vi "SetConfig.vi"(8 "error in (no error)":errorcluster, 11 "reference in":refnum<class "Barcode_Reader_Dialog.lvclass">) -> (0 "error out":errorcluster, 3 "reference out":refnum<class "Barcode_Reader_Dialog.lvclass">)   [LabVIEW 2022 SP3, in "Barcode_Reader_Dialog.lvlib" / "Barcode_Reader_Dialog.lvclass"]
uses:
  Barcode_Reader_Dialog.lvclass
  Components/Barcode_Reader_Base.lvlibp/Barcode_Reader_Base.lvclass
  C:/Projects/Medulla/ViPER/Examples/Flux_Capacitor_Tester/Components/ViPER.lvlibp/ViPER.lvclass
  Components/ViPER.lvlibp/ViPER.lvclass
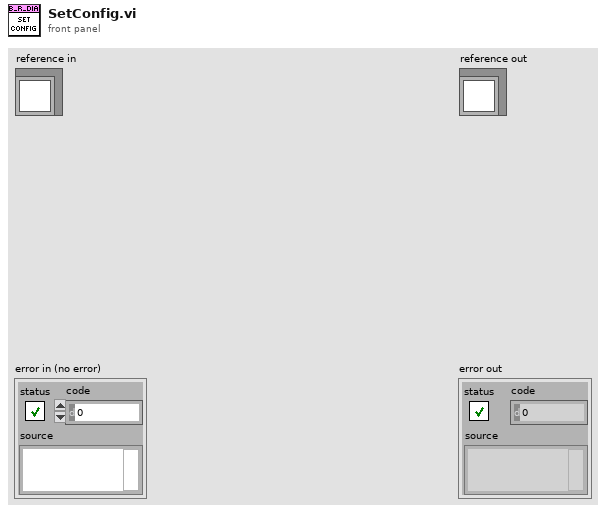
[diagram p1: front panel]
types:
  T1 = typedef "Barcode_Reader_Dialog.lvlib/Barcode_Reader_Dialog.lvclass/ObjectAttributes.ctl" = cluster{"Config":T2, "Serial":string}
  T2 = typedef "Barcode_Reader_Dialog.lvlib/Barcode_Reader_Dialog.lvclass/Config.ctl" = cluster{"default":string}
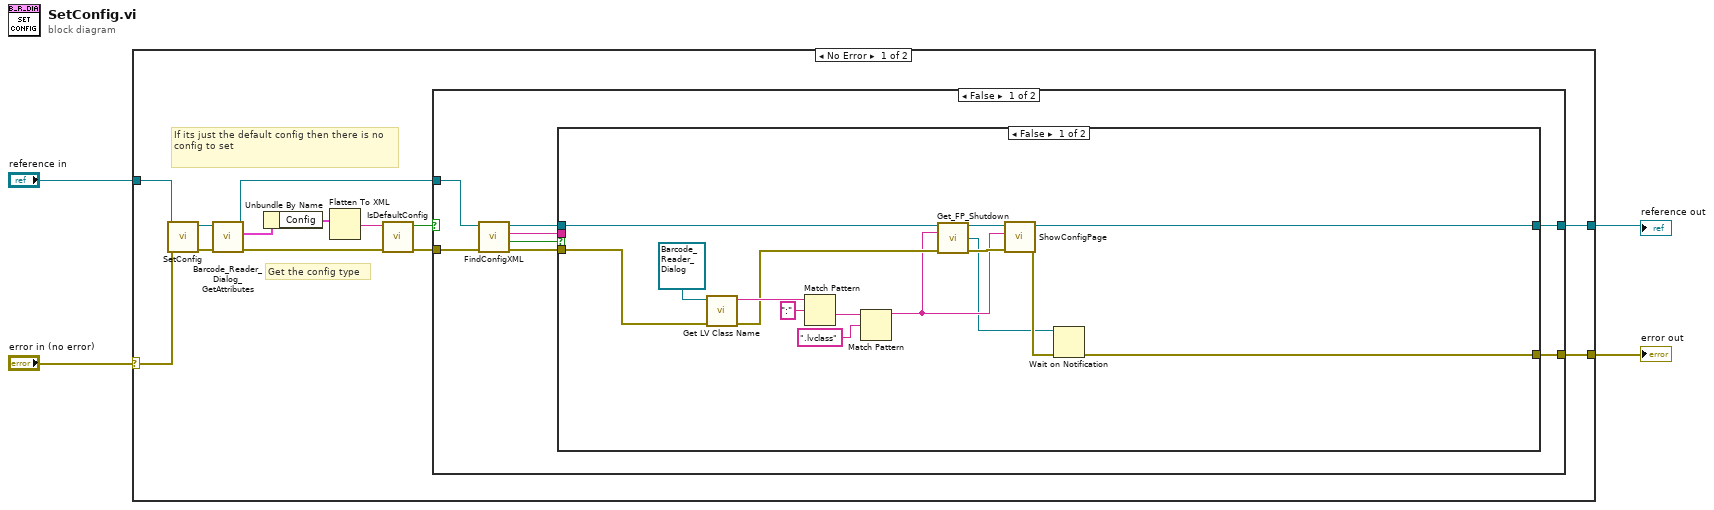
[diagram p0: block diagram]
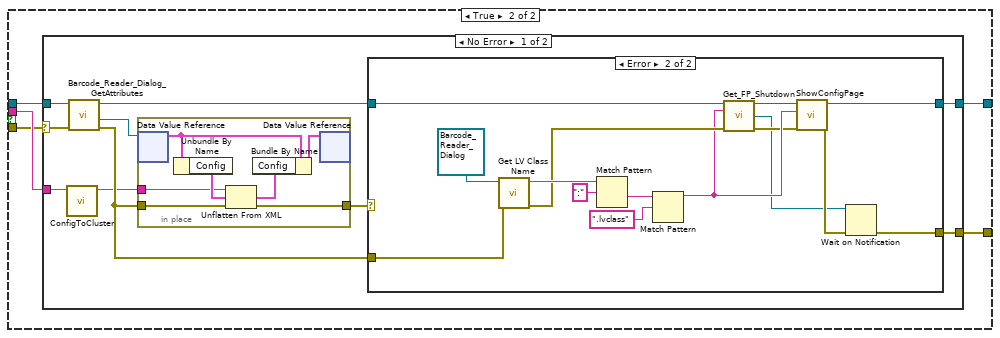
[diagram p2: hidden frame]
diagram:
  n1 = case shown="No Error" "error in (no error)" {
    selector: "error in (no error)" -> [w12 w85]
    tunnel: [w17 w85] -> w2
    tunnel: [w16 w84] -> w1
    tunnel: "reference in" -> [w10 w84]
    frame No Error {
      # "If its just the default config then there is no config to set"
      # "Get the config type"
      n2 = call-parent "SetConfig.vi"("error in (no error)"=w12, "reference in"=w10) -> ("error out"=w11:errorcluster, "reference out"=w9:refnum<class "Barcode_Reader_Dialog.lvclass">)  [unwired: 8 in]
      n3 = call "Barcode_Reader_Dialog_GetAttributes.vi"("error in (no error)"=w11, "reference in"=w9) -> ("error out"=w7:errorcluster, "Data"=w13:T1, "reference out"=w14:refnum<class "Barcode_Reader_Dialog.lvclass">)  [unwired: 6 in, 1 out]
      n4 = Unbundle By Name(w13) -> ("Config"=w15:T2)
      n5 = Flatten To XML(6:w15) -> (2:w8:string)
      n6 = call "IsDefaultConfig.vi"("error in (no error)"=w7, "Config XML"=w8) -> ("error out"=w6:errorcluster, "Is Default"=w5:bool)  [unwired: 8 in]
      n7 = case shown="False" w5 {
        tunnel: w6 -> [w23 w83]
        tunnel: w14 -> [w22 w82]
        tunnel: [w25 w83] -> w17
        tunnel: [w24 w82] -> w16
        frame False {
          n8 = call "FindConfigXML.vi"("error in (no error)"=w23, "Driver in"=w22) -> ("error out"=w18:errorcluster, "Exists?"=w19:bool, "Config XML"=w20:string, "Driver out"=w21:refnum<class "Barcode_Reader_Dialog.lvclass">)  [unwired: 6 in]
          n9 = case shown="False" w19 {
            tunnel: w20 -> [_ w43]
            tunnel: [w39 w45] -> w25
            tunnel: w18 -> [w32 w41]
            tunnel: w21 -> [w29 w42]
            tunnel: [w38 w44] -> w24
            frame False {
              n10 = call <vilib>:"Get LV Class Name.vi"("error in (no error)"=w32, "object"=refnum<class "Barcode_Reader_Dialog.lvclass"> refnum ("reference")) -> ("error out"=w31:errorcluster, "class name"=w36:string)  [unwired: 8 in]
              n11 = Match Pattern(string=w36, regular expression=":") -> (after substring=w34:string)  [unwired: 1 in, 3 out]
              n12 = Match Pattern(string=w34, regular expression=".lvclass") -> (before substring=w28:string)  [unwired: 1 in, 3 out]
              n13 = call "Get_FP_Shutdown.vi"("ViPER_Base in"=w29, "Ancestor"=w28, "error in (no error)"=w31) -> ("ViPER_Base out"=w27:refnum<class "Barcode_Reader_Dialog.lvclass">, "ConfigFP_Shutdown"=w26:refnum<notifier>, "error out"=w30:errorcluster)  [unwired: 9 in, 1 out]
              n14 = call-dynamic "ShowConfigPage.vi"("error in (no error)"=w30, "Ancestor"=w28, "Driver in"=w27) -> ("error out"=w40:errorcluster, "Driver out"=w38:refnum<class "Barcode_Reader_Dialog.lvclass">)  [unwired: 7 in]
              n15 = Wait on Notification(notifier=w26, error in (no error)=w40) -> (error out=w39:errorcluster)  [unwired: 2 in, 3 out]
            }
            frame True {
              n16 = case shown="No Error" w41 {
                selector: w41 -> [w53 w81]
                tunnel: [w55 w81] -> w45
                tunnel: [w54 w80] -> w44
                tunnel: w43 -> [w47 _]
                tunnel: w42 -> [w52 w80]
                frame No Error {
                  n17 = call "ConfigToCluster.vi"("Config XML"=w47) -> ("Cluster XML"=w46:string)  [unwired: 10 in]
                  n18 = call "Barcode_Reader_Dialog_GetAttributes.vi"("error in (no error)"=w53, "reference in"=w52) -> ("error out"=w48:errorcluster, "DataRef"=w51:refnum<data-value>, "reference out"=w50:refnum<class "Barcode_Reader_Dialog.lvclass">)  [unwired: 6 in, 1 out]
                  n19 = in-place {
                    in-place-border: w46 -> [w60]
                    in-place-border: w48 -> [w57]
                    in-place-border: [w56] -> w49
                    n20 = in-place-dvr #1(w51) -> (w62:T1)  [unwired: 1 out]
                    n21 = Unbundle By Name(w62) -> ("Config"=w61:T2)
                    n22 = Unflatten From XML(xml string=w60, type=w61, error in (no error)=w57) -> (value=w59:T2, error out=w56:errorcluster)
                    n23 = Bundle By Name(cluster=w62, "Config"=w59) -> (w58:T1)
                    n24 = in-place-dvr #1(w58) -> ()  [unwired: 2 out]
                  }
                  n25 = case shown="Error" w49 {
                    selector: w49 -> [w64 _]
                    tunnel: [w64 w73] -> w55
                    tunnel: w50 -> [w63 w69]
                    tunnel: [w63 w72] -> w54
                    tunnel: w48 -> [_ w71]
                    frame No Error {
                    }
                    frame Error {
                      n26 = call <vilib>:"Get LV Class Name.vi"("error in (no error)"=w71, "object"=refnum<class "Barcode_Reader_Dialog.lvclass"> refnum ("reference")) -> ("error out"=w70:errorcluster, "class name"=w77:string)  [unwired: 8 in]
                      n27 = Match Pattern(string=w77, regular expression=":") -> (after substring=w75:string)  [unwired: 1 in, 3 out]
                      n28 = Match Pattern(string=w75, regular expression=".lvclass") -> (before substring=w68:string)  [unwired: 1 in, 3 out]
                      n29 = call "Get_FP_Shutdown.vi"("ViPER_Base in"=w69, "Ancestor"=w68, "error in (no error)"=w70) -> ("ViPER_Base out"=w67:refnum<class "Barcode_Reader_Dialog.lvclass">, "ConfigFP_Shutdown"=w65:refnum<notifier>, "error out"=w66:errorcluster)  [unwired: 9 in, 1 out]
                      n30 = call-dynamic "ShowConfigPage.vi"("error in (no error)"=w66, "Ancestor"=w68, "Driver in"=w67) -> ("error out"=w79:errorcluster, "Driver out"=w72:refnum<class "Barcode_Reader_Dialog.lvclass">)  [unwired: 7 in]
                      n31 = Wait on Notification(notifier=w65, error in (no error)=w79) -> (error out=w73:errorcluster)  [unwired: 2 in, 3 out]
                    }
                  }
                }
                frame Error {
                }
              }
            }
          }
        }
        frame True {
        }
      }
    }
    frame Error {
    }
  }
  "error out" <- w2
  "reference out" <- w1
